vi "waveformchart.vi"() -> ()   [LabVIEW 2018]
panel:
  in  "?":bool
  in  "delay":dbl(slide) scale=0.0..2000.0
  out "Waveform Chart":dbl(graph)
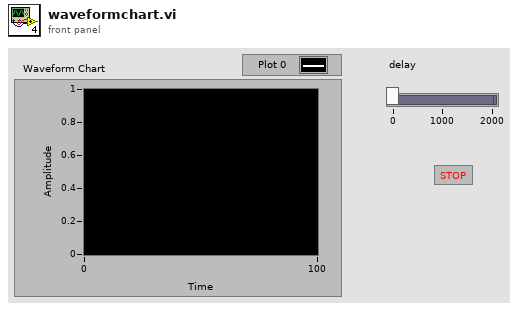
[diagram p1: front panel]
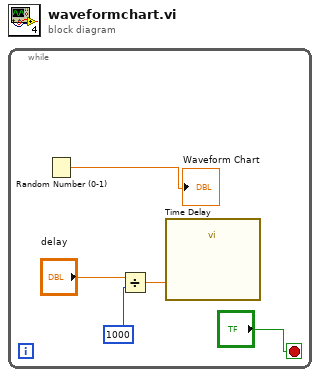
[diagram p0: block diagram]
diagram:
  n1 = while {
    stop <- "?" stop-if-true
    n2 = Random Number (0-1)() -> (number: 0 to 1=→"Waveform Chart":dbl)
    n3 = Divide(x="delay", y=1000) -> (x/y=w1:dbl)
    n4 = call "Time Delay"("Delay Time (s)"=w1) -> ()  [unwired: 10 in, 1 out]
  }
